vi "Simple PID Array.vi"(8 "D":dbl=0.05 format="%.2f", 9 "I":dbl=0.1 format="%.2f", 10 "P":dbl=1.0 format="%.2f", 11 "process variable":dbl[](array[numeric]) format="%.2f") -> (3 "output value":dbl[](array[numeric]) format="%.2f")   [LabVIEW 2016]
uses:
  <userlib>/_OpenG.lib/array/array.llb/Empty 1D Array (DBL)__ogtk.vi
panel:
  in  "upper limit":dbl=180.0 format="%.2f"
  in  "lower limit":dbl=-180.0 format="%.2f"
  in  "set point":dbl format="%.2f"
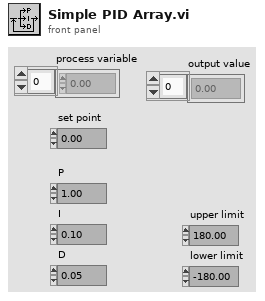
[diagram p1: front panel]
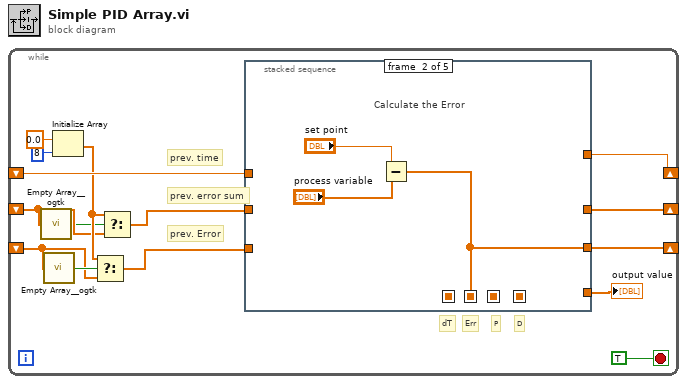
[diagram p0: block diagram]
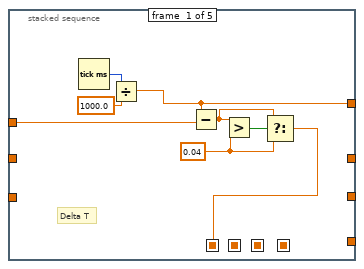
[diagram p2: hidden frame]
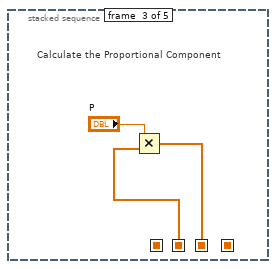
[diagram p3: hidden frame]
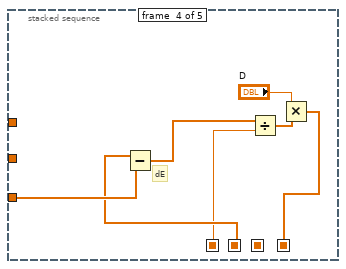
[diagram p4: hidden frame]
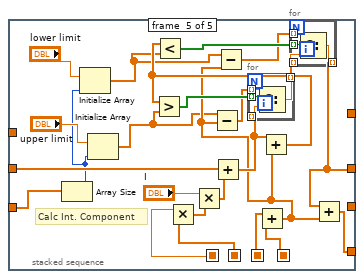
[diagram p5: hidden frame]
diagram:
  n1 = while {
    shift-left: _ -> [w6]
    shift-right: [w12] -> _
    shift-left: _ -> [w2]
    shift-right: [w13] -> _
    shift-left: _ -> [w14]
    shift-right: [w15] -> _
    stop <- TRUE stop-if-true
    # "dT"
    # "Err"
    # "D"
    # "P"
    # "prev. error sum"
    # "prev. time"
    # "prev. Error"
    n2 = call-poly <userlib>:"Empty Array__ogtk.vi"("Array"=w2) -> ("Empty Array?"=w1:bool)  [unwired: 8 in]
    n3 = call-poly <userlib>:"Empty Array__ogtk.vi"("Array"=w6) -> ("Empty Array?"=w7:bool)  [unwired: 8 in]
    n4 = Initialize Array(0.0 ("element"), 8 ("dimension size")) -> (w4:dbl[])
    n5 = Select(t=w4, s=w7, f=w6) -> (s? t:f=w5:dbl[])
    n6 = Select(t=w4, s=w1, f=w2) -> (s? t:f=w3:dbl[])
    n7 = stacked-sequence {
      seq-local: [w17 _ _ _ _] -> [_ _ _ w30 w58]
      seq-local: [_ w25 _ _ _] -> [_ _ w28 w35 w59]
      seq-local: [_ _ w27 _ _] -> [_ _ _ _ w54]
      seq-local: [_ _ _ w31 _] -> [_ _ _ _ w53]
      tunnel: [w20 _ _ _ _] -> w15
      tunnel: w14 -> [w23 _ _ _ _]
      tunnel: w3 -> [_ _ _ _ w60]
      tunnel: [_ _ _ _ w47] -> w13
      tunnel: [_ w25 _ _ _] -> w12
      tunnel: w5 -> [_ _ _ w36 w38]
      tunnel: [_ _ _ _ w51] -> w10
      frame #0 {
        w16 = 0.04
        # "Delta T"
        n8 = Tick Count (ms)() -> (millisecond timer value=w21:u32)
        n9 = Divide(x=w21, y=1000.0) -> (x/y=w20:dbl)
        n10 = Subtract(x=w20, y=w23) -> (x-y=w18:dbl)
        n11 = Greater?(x=w18, y=w16) -> (0:w19:bool)
        n12 = Select(t=w18, s=w19, f=w16) -> (s? t:f=w17:dbl)
      }
      frame #1 {
        # "Calculate the Error"
        n13 = Subtract(x="set point", y="process variable") -> (x-y=w25:dbl[])
      }
      frame #2 {
        # "Calculate the Proportional Component"
        n14 = Multiply(x="P", y=w28) -> (x*y=w27:dbl[])
      }
      frame #3 {
        # "dE"
        n15 = Subtract(x=w35, y=w36) -> (x-y=w34:dbl[])
        n16 = Divide(x=w34, y=w30) -> (x/y=w33:dbl[])
        n17 = Multiply(x="D", y=w33) -> (x*y=w31:dbl[])
      }
      frame #4 {
        # "Calc Int. Component"
        n18 = Array Size(array=w38) -> (size(s)=w37:i32)
        n19 = Initialize Array("lower limit", w37) -> (w41:dbl[])
        n20 = Initialize Array("upper limit", w37) -> (w39:dbl[])
        n21 = Multiply(x=w58, y=w59) -> (x*y=w57:dbl[])
        n22 = Multiply(x="I", y=w57) -> (x*y=w55:dbl[])
        n23 = Add(x=w60, y=w55) -> (x+y=w49:dbl[])
        n24 = Add(x=w54, y=w53) -> (x+y=w43:dbl[])
        n25 = Subtract(x=w39, y=w43) -> (x-y=w45:dbl[])
        n26 = Subtract(x=w41, y=w43) -> (x-y=w44:dbl[])
        n27 = Add(x=w49, y=w43) -> (x+y=w46:dbl[])
        n28 = Greater?(x=w46, y=w39) -> (0:w52:bool[])
        n29 = Less?(x=w46, y=w41) -> (x < y?=w50:bool[])
        n30 = for {
          tunnel: w52 -> [w68] mode=indexing
          tunnel: w49 -> [w67] mode=indexing
          tunnel: [w66] -> w48 mode=indexing
          tunnel: w45 -> [w65] mode=indexing
          n31 = Select(t=w65, s=w68, f=w67) -> (s? t:f=w66:dbl)
        }
        n32 = for {
          tunnel: w50 -> [w64] mode=indexing
          tunnel: w48 -> [w63] mode=indexing
          tunnel: [w62] -> w47 mode=indexing
          tunnel: w44 -> [w61] mode=indexing
          n33 = Select(t=w61, s=w64, f=w63) -> (s? t:f=w62:dbl)
        }
        n34 = Add(x=w47, y=w43) -> (x+y=w51:dbl[])
      }
    }
    "output value" <- w10
  }
